vi "DataProcessor.vi"(3 "PumpOffBkgd":dbl[](array[numeric]), 4 "PumpOnBkgd":dbl[](array[numeric]), 5 "Data":dbl[][](array[numeric]), 6 "# of Images":u16) -> (0 "PumpOff":dbl[](array[numeric]), 1 "PumpOn":dbl[](array[numeric]), 2 "Raman":dbl[](array[numeric]))   [LabVIEW 2013]
panel:
  # "This vi takes the Data from the DataGrabber.vi and processes it splitting up the Raman Pump On and Off spectra as well as creating the Raman Gain Spectrum"
  # "Data Output"
  # "Data Input"
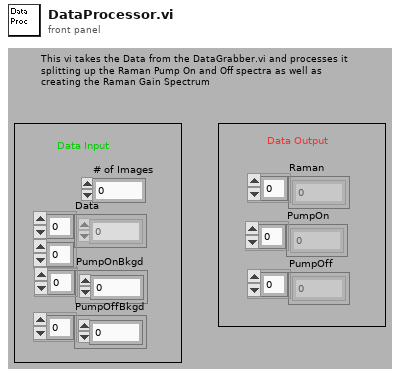
[diagram p1: front panel]
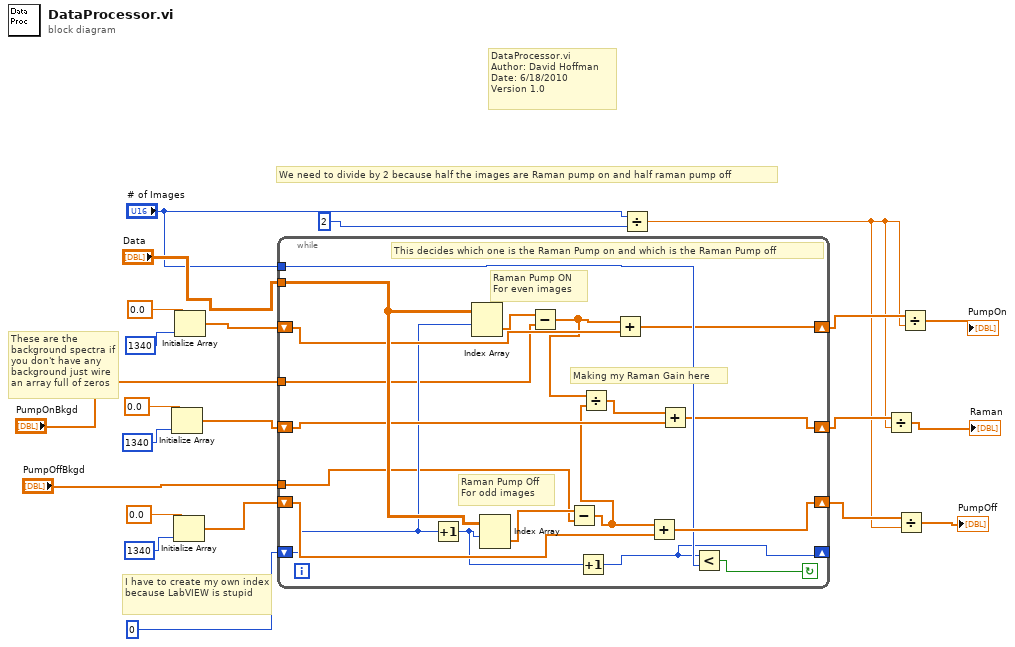
[diagram p0: block diagram]
diagram:
  # "These are the background spectra if you don't have any background just wire an array full of zeros"
  # "I have to create my own index because LabVIEW is stupid"
  # "We need to divide by 2 because half the images are Raman pump on and half raman pump off"
  # "DataProcessor.vi\nAuthor: David Hoffman\nDate: 6/18/2010\nVersion 1.0"
  n1 = Initialize Array(0.0, u32 1340) -> (w7:dbl[])
  n2 = Initialize Array(0.0, u32 1340) -> (w17:dbl[])
  n3 = Initialize Array(0.0, u32 1340) -> (w18:dbl[])
  n4 = while {
    tunnel: "Data" -> [w39]
    shift-right: [w36] -> w16
    shift-left: w18 -> [w38]
    shift-right: [w40] -> w15
    shift-left: w17 -> [w41]
    tunnel: "# of Images" -> [w37]
    shift-right: [w34] -> w6
    shift-left: w7 -> [w33]
    shift-right: [w29] -> _
    shift-left: 0 -> [w31]
    tunnel: "PumpOnBkgd" -> [w27]
    tunnel: "PumpOffBkgd" -> [w24]
    stop <- w32 continue-if-true
    # "Making my Raman Gain here"
    # "Raman Pump ON\nFor even images"
    # "Raman Pump Off\nFor odd images"
    # "This decides which one is the Raman Pump on and which is the Raman Pump off"
    n5 = Increment(x=w31) -> (x+1=w30:i32)
    n6 = Index Array(array=w39, index (row)=w31) -> (element=w28:dbl[])  [unwired: 1 in]
    n7 = Index Array(array=w39, index (row)=w30) -> (element=w25:dbl[])  [unwired: 1 in]
    n8 = Subtract(x=w28, y=w27) -> (x-y=w26:dbl[])
    n9 = Subtract(x=w25, y=w24) -> (x-y=w23:dbl[])
    n10 = Increment(x=w30) -> (x+1=w29:i32)
    n11 = Divide(x=w26, y=w23) -> (x/y=w35:dbl[])
    n12 = Add(x=w26, y=w38) -> (x+y=w36:dbl[])
    n13 = Add(x=w23, y=w41) -> (x+y=w40:dbl[])
    n14 = Add(x=w35, y=w33) -> (x+y=w34:dbl[])
    n15 = Less?(x=w29, y=w37) -> (x < y?=w32:bool)
  }
  n16 = Divide(x="# of Images", y=2) -> (x/y=w5:dbl)
  n17 = Divide(x=w6, y=w5) -> (x/y=→"Raman":dbl[])
  n18 = Divide(x=w15, y=w5) -> (x/y=→"PumpOff":dbl[])
  n19 = Divide(x=w16, y=w5) -> (x/y=→"PumpOn":dbl[])
